vi "Adquirir Parametro del Generador por Modbus.vi"(8 "error in":errorcluster, 10 "VISA resource name":refnum<visa-resource-name>, 11 "queue":refnum<queue>) -> (0 "error out":errorcluster, 1 "Ring_Gen_Out":i32=2, 2 "Pot_gen_out":dbl, 3 "Time_gen":timestamp, 4 "Flujo_Gen_Out":bool, 5 "queue out":refnum<queue>)   [LabVIEW 2015]
uses:
  Application/ClusterM2.ctl
  Login Window Control Folder/global variable.vi
panel:
  # "HOLDING REGISTER\n\nA) 201 > BATERIA\nB) 102 >  FACTOR DE POTENCIA\n\n*EL LISTADO DE LOS HOLDING REGISTERS SE ENCUENTRA EN ARCHIVO EMPC 4 Modbus Registers 4.2 Prod Software"
  # "SCALLING\n\nFORMULA APLICADA AL VALOR ALMACENADO EN EL HOLDING REGISTER\n\nA) 0.05\n\nB) 1/16384 _ 0,00006103515623\n\n* SE ENCUENTRA EN ARCHIVO EMPC 4 Modbus Registers 4.2 Prod Software - Columna Scaling Resolution"
  # "OFFSET\n\nA) 0\n\nB) -1,0\n\n\n SE ENCUENTRA EN ARCHIVO EMPC 4 Modbus Registers 4.2 Prod Software - Columna Offset"
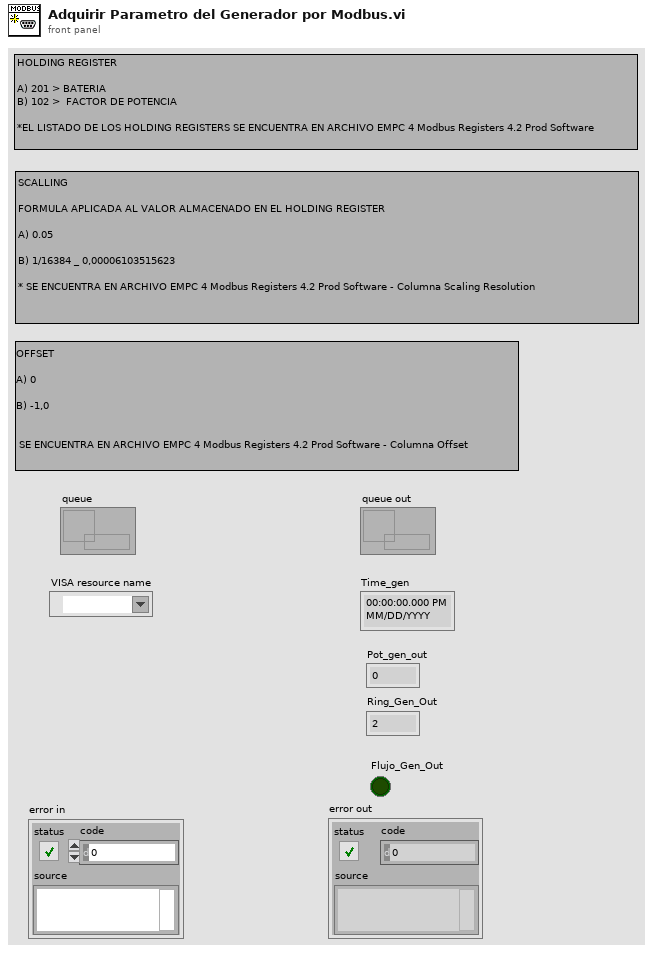
[diagram p1: front panel]
types:
  T1 = typedef "ClusterM2.ctl" = cluster{"timeStamp":timestamp, "Data":dbl[], "group":string}
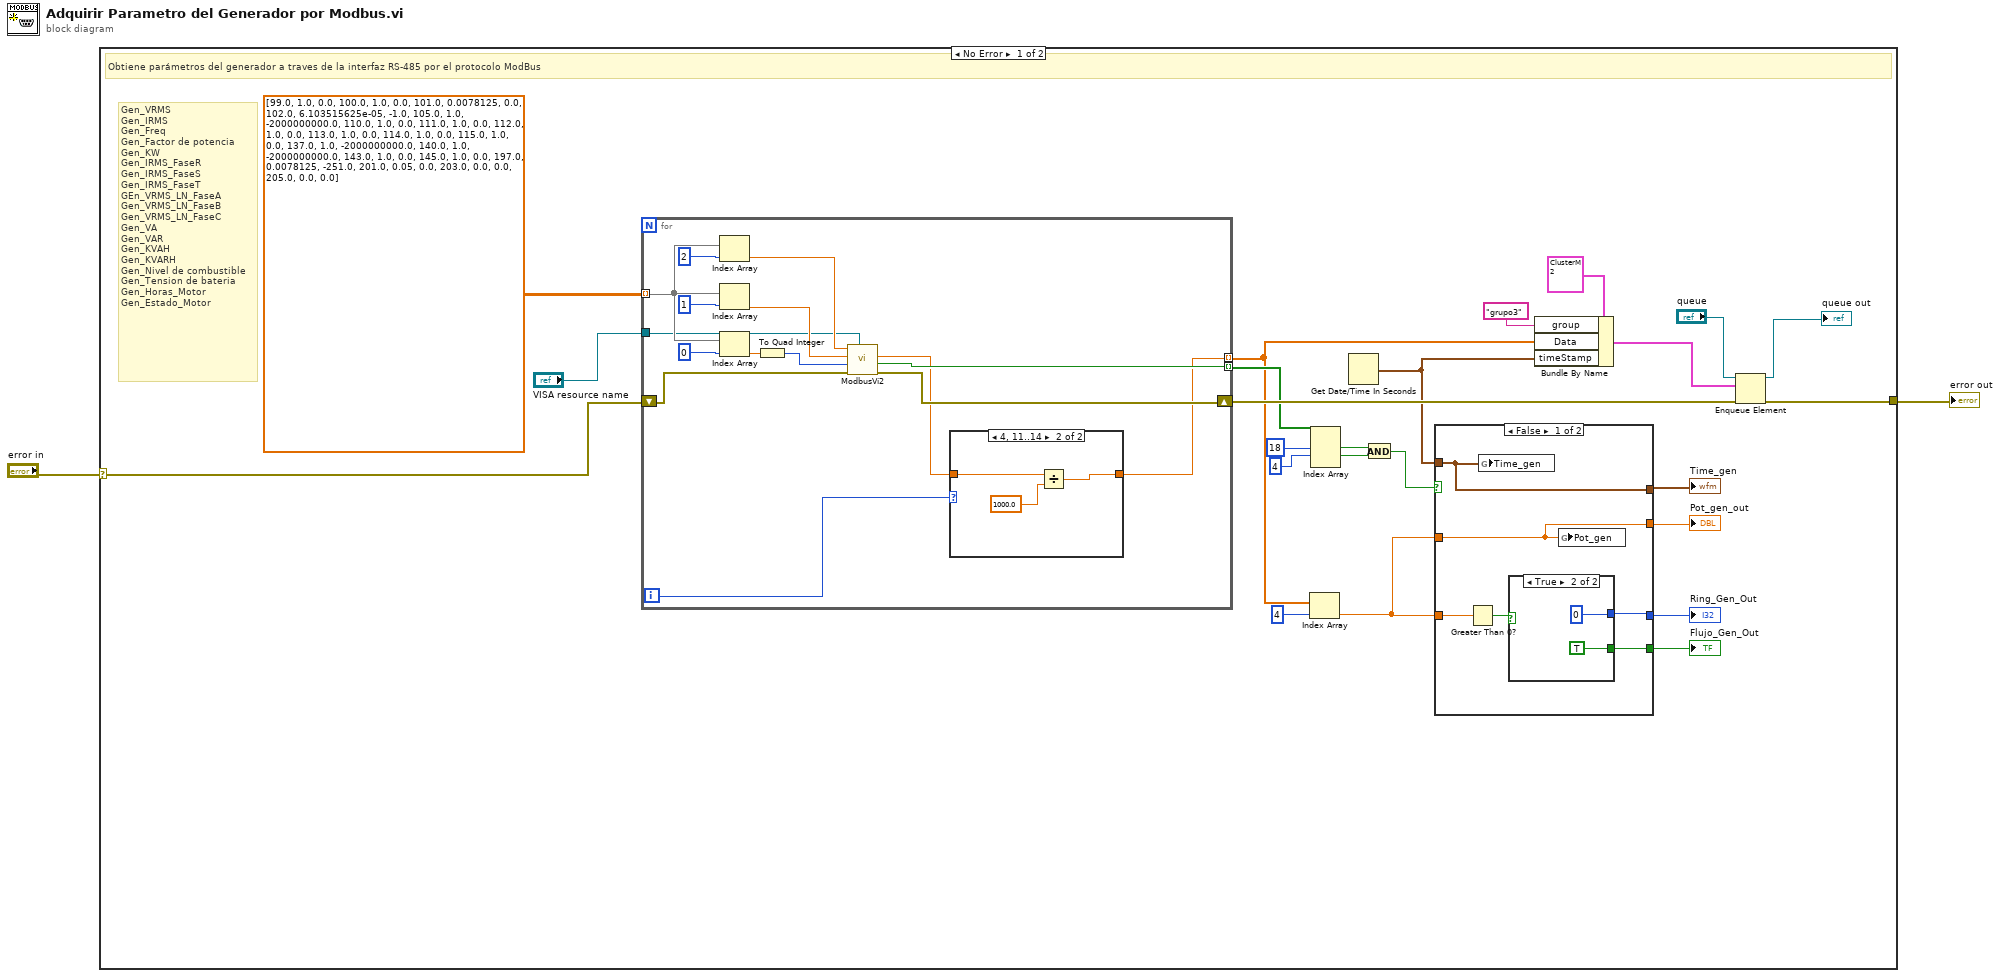
[diagram p0: block diagram]
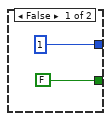
[diagram p2: hidden frame]
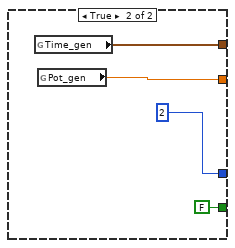
[diagram p3: hidden frame]
diagram:
  n1 = case shown="No Error" "error in" {
    selector: "error in" -> [w5 w60]
    tunnel: [w6 w60] -> w1
    frame No Error {
      # "Gen_VRMS\nGen_IRMS\nGen_Freq\nGen_Factor de potencia\nGen_KW\nGen_IRMS_FaseR\nGen_IRMS_FaseS\nGen_IRMS_FaseT\nGEn_VRMS_LN_FaseA\nGen_VRMS_LN_FaseB\nGen_VRMS_LN_FaseC\nGen_VA\nGen_VAR\nGen_KVAH\nGen_KVARH\nGen_Nivel de combustible\nGen_Tension de bateria\nGen_Horas_Motor\nGen_Estado_Motor"
      # "Obtiene parámetros del generador a traves de la interfaz RS-485 por el protocolo ModBus"
      n2 = for {
        tunnel: dbl[][] [[99.0, 1.0, 0.0], [100.0, 1.0, 0.0], [101.0, 0.0078125, 0.0], [102.0, 6.103515625e-05, -1.0], [105.0, 1.0, -2000000000.0], [110.0, 1.0, 0.0], [111.0, 1.0, 0.0], [112.0, 1.0, 0.0], [113.0, 1.0, 0.0], [114.0, 1.0, 0.0], [115.0, 1.0, 0.0], [137.0, 1.0, -2000000000.0], [140.0, 1.0, -2000000000.0], [143.0, 1.0, 0.0], [145.0, 1.0, 0.0], [197.0, 0.0078125, -251.0], [201.0, 0.05, 0.0], [203.0, 0.0, 0.0], [205.0, 0.0, 0.0]] ("Entradas") -> [w55] mode=indexing
        tunnel: "VISA resource name" -> [w45]
        shift-right: [w48] -> w19
        shift-left: w5 -> [w44]
        tunnel: [w41] -> w3 mode=indexing
        tunnel: [w46] -> w16 mode=indexing
        i -> [w43]
        n3 = Index Array(array=w55, index=2) -> (element=w47:dbl)
        n4 = Index Array(array=w55, index=1) -> (element=w50:dbl)
        n5 = Index Array(array=w55, index=0) -> (element=w52:dbl)
        n6 = To Quad Integer(1:w52) -> (0:w49:i64)
        n7 = call "ModbusVi2.vi"("VISA resource name"=w45, "error in"=w44, "Holding Register"=w49, "Scalling"=w50, "Offset"=w47) -> ("error out"=w48:errorcluster, "error de conexion"=w46:bool, "Value"=w42:dbl)  [unwired: 3 in, 1 out]
        n8 = case shown="4, 11..14" w43 {
          tunnel: w42 -> [w56 w59]
          tunnel: [w56 w57] -> w41
          frame 0, Default {
          }
          frame 4, 11..14 {
            n9 = Divide(x=w59, y=1000.0) -> (x/y=w57:dbl)
          }
        }
      }
      n10 = Index Array(array=w3, index=4) -> (element=w11:dbl)
      n11 = Index Array(array=w16, index #1=18 ("index"), index #2=4 ("index")) -> (element #1=w13:bool, element #2=w9:bool)  [unwired: 1 in, 1 out]
      n12 = Get Date/Time In Seconds() -> (seconds since 1Jan1904=w4:timestamp)
      n13 = And(x=w13, y=w9) -> (x .and. y?=w8:bool)
      n14 = case shown="False" w8 {
        tunnel: w4 -> [w32 _]
        tunnel: [w32 w40] -> w17
        tunnel: w11 -> [w27 _]
        tunnel: [w27 w39] -> w14
        tunnel: [w31 2] -> w12
        tunnel: w11 -> [w29 _]
        tunnel: [w30 FALSE] -> w7
        frame False {
          n15 = Greater Than 0?(x=w29) -> (x > 0?=w28:bool)
          n16 = global write "global variable.vi" "Time_gen"(w32) -> ()
          n17 = case shown="True" w28 {
            tunnel: [1 0] -> w31
            tunnel: [FALSE TRUE] -> w30
            frame False {
            }
            frame True {
            }
          }
          n18 = global write "global variable.vi" "Pot_gen"(w27) -> ()
        }
        frame True {
          n19 = global read "global variable.vi" "Time_gen"() -> (w40:timestamp)
          n20 = global read "global variable.vi" "Pot_gen"() -> (w39:dbl)
        }
      }
      "Time_gen" <- w17
      "Pot_gen_out" <- w14
      "Ring_Gen_Out" <- w12
      "Flujo_Gen_Out" <- w7
      n21 = Bundle By Name(cluster=T1 {"timeStamp"=timestamp(0 s since 1904-01-01), "Data"=[], "group"=""} ("M2"), "group"="grupo3" ("grupo"), "Data"=w3, "timeStamp"=w4) -> (w22:T1)
      n22 = Enqueue Element(queue="queue", element=w22, error in (no error)=w19) -> (queue out=→"queue out":refnum<queue>, error out=w6:errorcluster)  [unwired: 1 in, 1 out]
    }
    frame Error {
    }
  }
  "error out" <- w1
